vi "hydraharp_normalize_correlation.vi"(8 "error in (no error)":errorcluster, 11 "hydraharp.lvclass":refnum<class "hydraharp.lvclass">) -> (0 "error out":errorcluster, 3 "hydraharp.lvclass 2":refnum<class "hydraharp.lvclass">)   [LabVIEW 2015, in "hydraharp.lvclass"]
uses:
  hydraharp.lvclass
  hydraharp.lvclass/hydraharp.ctl
panel:
  out "x-y":dbl
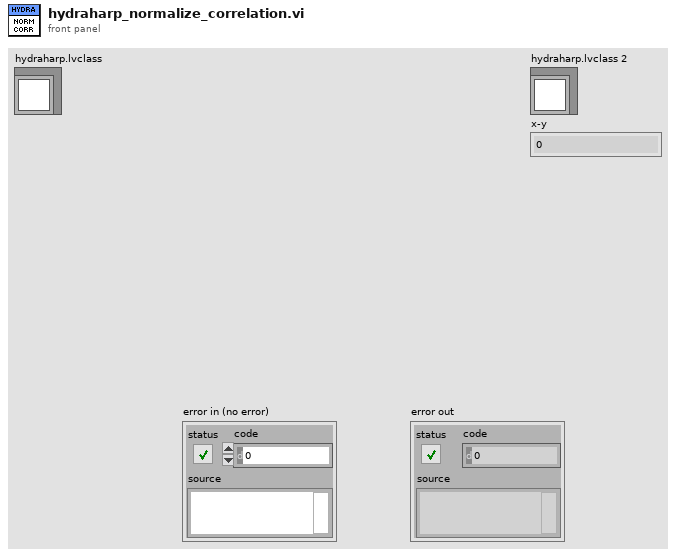
[diagram p1: front panel]
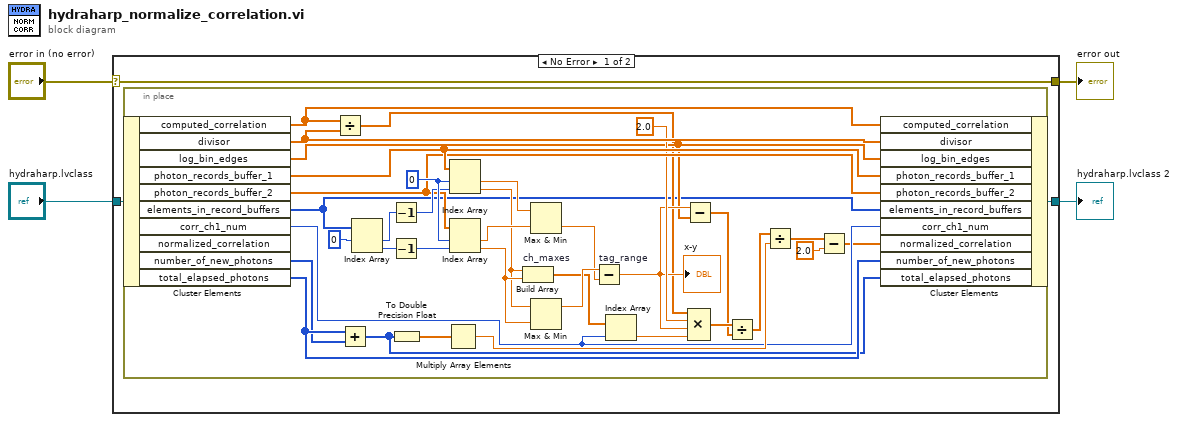
[diagram p0: block diagram]
diagram:
  n1 = case shown="No Error" "error in (no error)" {
    selector: "error in (no error)" -> [w5 w44]
    tunnel: "hydraharp.lvclass" -> [w7 w43]
    tunnel: [w6 w43] -> w2
    tunnel: [w5 w44] -> w1
    frame No Error {
      n2 = in-place {
        w42 = 0 ("index")
        n3 = in-place-cluster #1(w7) -> ("computed_correlation"=w13:dbl[], "divisor"=w32:dbl[], "log_bin_edges"=w22:dbl[], "photon_records_buffer_1"=w34:dbl[], "photon_records_buffer_2"=w33:dbl[], "elements_in_record_buffers"=w11:i32[], "corr_ch1_num"=w17:i32, "number_of_new_photons"=w9:i32[], "total_elapsed_photons"=w10:i32[])  [unwired: 1 out]
        n4 = Divide(x=w13, y=w32) -> (x/y=w20:dbl[])
        n5 = Add(x=w10, y=w9) -> (x+y=w8:i32[])
        n6 = Index Array(array=w11, index #1=0 ("index")) -> (element #1=w26:i32, element #2=w25:i32)  [unwired: 1 in]
        n7 = Decrement(x=w26) -> (x-1=w39:i32)
        n8 = Decrement(x=w25) -> (x-1=w40:i32)
        n9 = To Double Precision Float(number=w8) -> (double precision float=w12:dbl[])
        n10 = Multiply Array Elements(1:w12) -> (0:w18:dbl)
        n11 = Index Array(array=w34, index #1=w42, index #2=w39) -> (element #1=w37:dbl, element #2=w30:dbl)
        n12 = Index Array(array=w33, index #1=w42, index #2=w40) -> (element #1=w38:dbl, element #2=w31:dbl)
        n13 = Build Array "ch_maxes"(w30, w31) -> (w29:dbl[])
        n14 = Max & Min(x=w37, y=w38) -> (min(x,y)=w35:dbl)  [unwired: 1 out]
        n15 = Max & Min(x=w30, y=w31) -> (max(x,y)=w36:dbl)  [unwired: 1 out]
        n16 = Subtract "tag_range"(x=w36, y=w35) -> (x-y=w23:dbl)
        "x-y" <- w23
        n17 = Index Array(array=w29, index=w17) -> (element=w27:dbl)
        n18 = Subtract(x=w23, y=w22) -> (x-y=w21:dbl[])
        n19 = Compound Arithmetic op=MULTIPLY(w20, 2.0, w23, w27) -> (w24:dbl[])
        n20 = Divide(x=w24, y=w21) -> (x/y=w19:dbl[])
        n21 = Divide(x=w19, y=w18) -> (x/y=w16:dbl[])
        n22 = Subtract(x=w16, y=2.0) -> (x-y=w14:dbl[])
        n23 = in-place-cluster #1("computed_correlation"=w13, "divisor"=w32, "log_bin_edges"=w22, "photon_records_buffer_1"=w34, "photon_records_buffer_2"=w33, "elements_in_record_buffers"=w11, "corr_ch1_num"=w17, "normalized_correlation"=w14, "number_of_new_photons"=w10, "total_elapsed_photons"=w8) -> (w6:refnum<class "hydraharp.lvclass">)
      }
    }
    frame Error {
    }
  }
  "error out" <- w1
  "hydraharp.lvclass 2" <- w2
